vi "LabVIEW JSON Example Modify.vi"() -> ()   [LabVIEW 2019]
uses:
  lib/Element Type.ctl
  lib/Element Set Behavior.ctl
  lib/labview_json.lvlib
panel:
  in  "Values":cluster{"powers":string[], "age":i32}={"powers"=["earth", "fire", "wind", "water"], "age"=89}
  out "JSON out 2":string
  out "Exists? 4":bool
  out "error out 4":errorcluster
  in  "Behavior (Add or Modify)":T1
  out "JSON out":string
  out "Exists? 3":bool
  out "Value 2":variant
  out "error out 3":errorcluster
  out "Value":variant
  out "Exists? 2":bool
  out "error out 2":errorcluster
  out "Type":T2
  out "Exists?":bool
  out "Keys/Indexes":string[](array[string])
  out "error out":errorcluster
  in  "JSON in":string="{\n  \"squadName\": \"Super hero squad\",\n  \"homeTown\": \"Metro City\",\n  \"formed\": 2016,\n  \"secretBase\": \"Super tower\",\n  \"active\": true,\n  \"members\": [\n    {\n      \"name\": \"Molecule Man\",\n      \"age\": 29,\n      \"secretIdentity\": \"Dan Jukes\",\n      \"powers\": [\n        \"Radiation resistance\",\n        \"Turning tiny\",\n        \"Radiation blast\"\n      ]\n    },\n    {\n      \"name\": \"Madame Uppercut\",\n      \"age\": 39,\n      \"secretIdentity\": \"Jane Wilson\",\n      \"powers\": [\n        \"Million tonne punch\",\n        \"Damage resistance\",\n        \"Superhuman reflexes\"\n      ]\n    },\n    {\n      \"name\": \"Eternal Flame\",\n      \"age\": 1000000,\n      \"secretIdentity\": \"Unknown\",\n      \"powers\": [\n        \"Immortality\",\n        \"Heat Immunity\",\n        \"Inferno\",\n        \"Teleportation\",\n        \"Interdimensional travel\"\n      ]\n    }\n  ]\n}"
  in  "Root Path ([]=Root)":string[](array[string])=["members", "0"]
  # "1. Specify nested path"
  # "2. List elements"
  # "3. Get element"
  # "4. Pop element"
  # "5. Set element"
  # "Behavior Options:\n    Add or Modify - Create or modify elements (Arrays resize)\n    Modify - Modify elements only if exists (Arrays don't resize)\n    Replace - Replace elements (Root paths excepted)"
  # "Objects = Key\nArrays = Index"
  # "A root path is the nested \nobject key or array index\nto the element you want\nto list, get, pop or set."
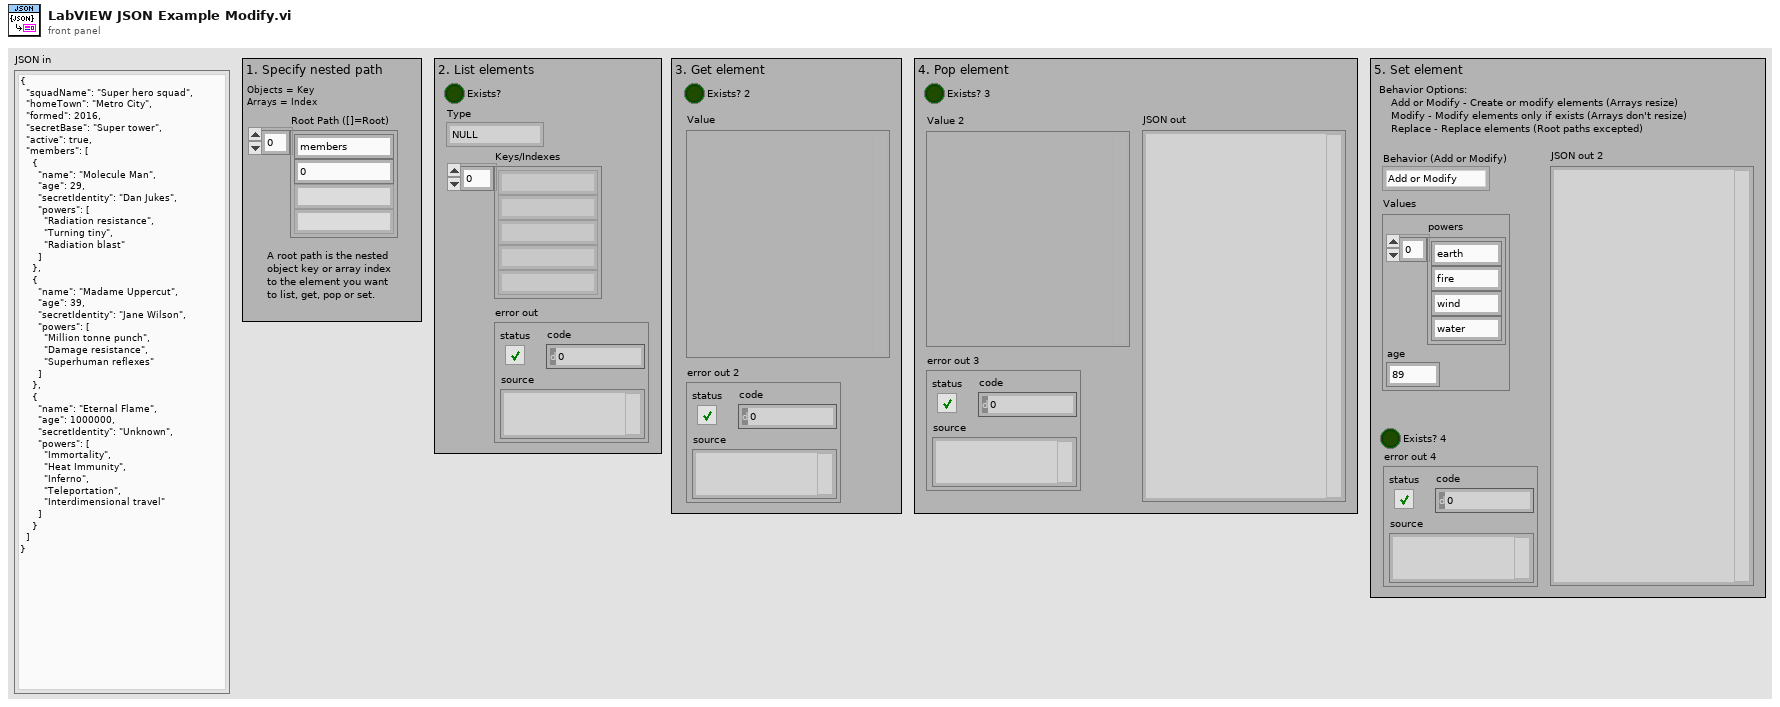
[diagram p1: front panel]
types:
  T1 = typedef "labview_json.lvlib/Element Set Behavior.ctl" = enum8{"Add or Modify", "Modify Only", "Replace"}
  T2 = typedef "labview_json.lvlib/Element Type.ctl" = enum8{"NULL", "OBJECT", "ARRAY", "BOOL", "INT", "UINT", "FLOAT", "STRING"}
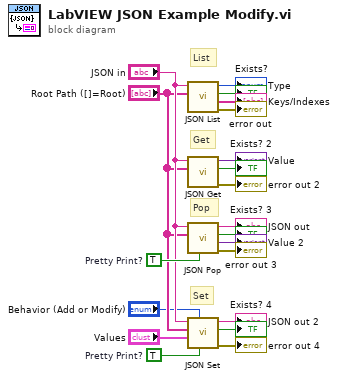
[diagram p0: block diagram]
diagram:
  w6 = TRUE  # Pretty Print?
  w9 = TRUE  # Pretty Print?
  # "Set"
  # "Pop"
  # "Get"
  # "List"
  n1 = call "JSON List.vi"("Root Path ([]=Root)"="Root Path ([]=Root)", "JSON in"="JSON in") -> ("error out"=→"error out":errorcluster, "Keys/Indexes"=→"Keys/Indexes":string[], "Exists?"=→"Exists?":bool, "Type"=→"Type":T2)  [unwired: 6 in]
  n2 = call "JSON Get.vi"("Root Path ([]=Root)"="Root Path ([]=Root)", "JSON in"="JSON in") -> ("error out"=→"error out 2":errorcluster, "Exists?"=→"Exists? 2":bool, "Value"=→"Value":variant)  [unwired: 7 in]
  n3 = call "JSON Pop.vi"("Pretty Print? (F)"=w9, "Root Path ([]=Root)"="Root Path ([]=Root)", "JSON in"="JSON in") -> ("error out"=→"error out 3":errorcluster, "Value"=→"Value 2":variant, "Exists?"=→"Exists? 3":bool, "JSON out"=→"JSON out":string)  [unwired: 5 in]
  n4 = call "JSON Set.vi"("Pretty Print? (F)"=w6, "Behavior (Add or Modify)"="Behavior (Add or Modify)", "Value"="Values", "Root Path ([]=Root)"="Root Path ([]=Root)", "JSON in"="JSON in") -> ("error out"=→"error out 4":errorcluster, "Exists?"=→"Exists? 4":bool, "JSON out"=→"JSON out 2":string)  [unwired: 4 in]
